vi "WPI_RobotDriveOpen7MotorWithSPARK.vi"(0 "Left Lead Motor":T1=enum."Invalid", 1 "Left Motor Inverted":bool, 5 "Left Follower Motor":T1=enum."Invalid", 7 "Front Left Motor":T1=enum."Invalid", 9 "Front Right Motor":T1=enum."Invalid", 12 "Front Left Motor Inverted":bool) -> (4 "RobotDriveDevRef":T2={"DevStatus"={"status"=FALSE, "code"=0, "source"=""}, "Motors[]"=[], "Square Inputs"=FALSE, "Max Output"=1.0}, 15 "error out":errorcluster)   [LabVIEW 2018]
doc: "Opens a reference to the robot drive for a four-motor robot using Rev Robotics SPARK motor controllers.\n\nThis software is licensed. Open the labview\\readme\\WPI Robotics Library Open Source License.txt file for more information."
uses:
  <vilib>/Rock Robotics/WPI/SafetyOutput/WPI_SafetyOutputConfigMenu.ctl
  <vilib>/Rock Robotics/WPI/RobotDrive/WPI_RobotDriveOpen2MotorWithExistingMotors.vi
  <vilib>/Rock Robotics/WPI/RobotDrive/WPI_RobotDriveDevRef.ctl
  <vilib>/Rock Robotics/WPI/MotorControl/WPI_MotorControlDeviceRef.ctl
  <vilib>/Rock Robotics/SystemInterfaces/DIO/FPGA_DIOChannel.ctl
  <vilib>/Rock Robotics/SystemInterfaces/DIO/FPGA_DIOPWMChannel.ctl
  <vilib>/Rock Robotics/WPI/PWM/WPI_PWMDeadband.ctl
  <vilib>/Rock Robotics/WPI/MotorControl/WPI_MotorControlType.ctl
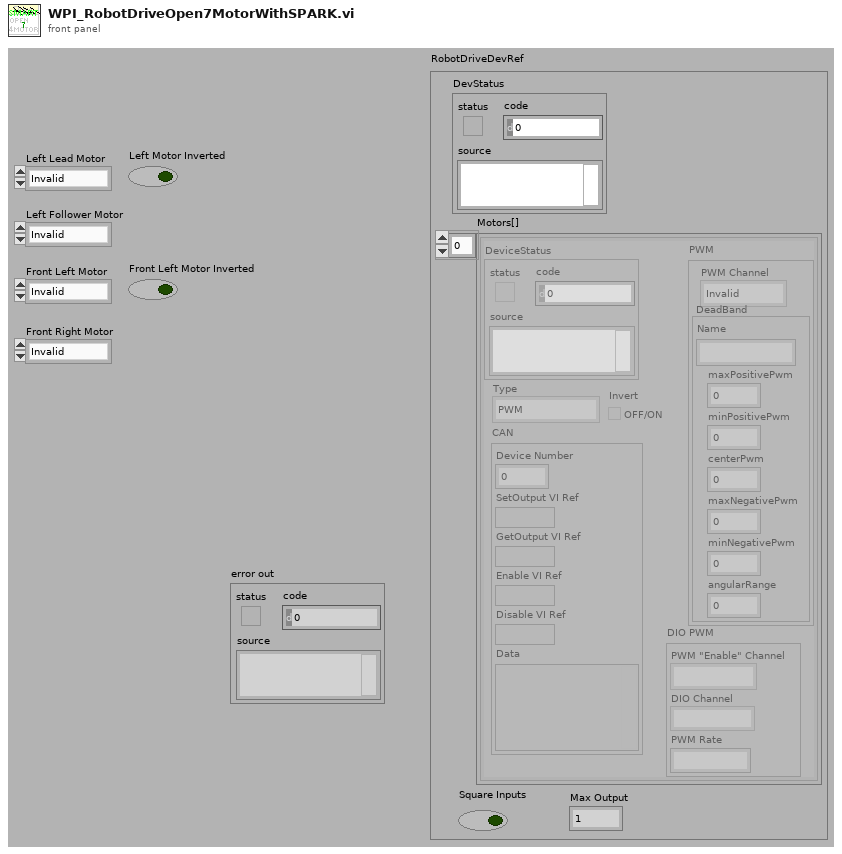
[diagram p1: front panel]
types:
  T1 = typedef "FPGA_DIOPWMChannel.ctl" = enum8{"PWM 0", "PWM 1", "PWM 2", "PWM 3", "PWM 4", "PWM 5", "PWM 6", "PWM 7", "PWM 8", "PWM 9", "PWM MXP 0", "PWM MXP 1", "PWM MXP 2", "PWM MXP 3", "PWM MXP 4", "PWM MXP 5", "PWM MXP 6", "PWM MXP 7", "PWM MXP 8", "PWM MXP 9", "Invalid"}
  T2 = typedef "WPI_RobotDriveDevRef.ctl" = cluster{"DevStatus":errorcluster, "Motors[]":T3[], "Square Inputs":bool, "Max Output":dbl}
  T3 = typedef "WPI_MotorControlDeviceRef.ctl" = cluster{"DeviceStatus":errorcluster, "Type":T4, "PWM":cluster{"PWM Channel":T1, "DeadBand":T5}, "CAN":cluster{"Device Number":u8, "SetOutput VI Ref":variant, "GetOutput VI Ref":variant, "Enable VI Ref":variant, "Disable VI Ref":variant, "Data":variant}, "Invert":bool, "DIO PWM":cluster{"PWM \"Enable\" Channel":T1, "DIOChannel":T6, "PWM Rate":dbl}}
  T4 = typedef "WPI_MotorControlType.ctl" = enum16{"PWM", "CAN", "DIO PWM"}
  T5 = typedef "WPI_PWMDeadband.ctl" = cluster{"Name":string, "maxPositivePwm":i32, "minPositivePwm":i32, "centerPwm":i32, "maxNegativePwm":i32, "minNegativePwm":i32, "angularRange":u16}
  T6 = typedef "FPGA_DIOChannel.ctl" = enum8{"DIO 0", "DIO 1", "DIO 2", "DIO 3", "DIO 4", "DIO 5", "DIO 6", "DIO 7", "DIO 8", "DIO 9", "DIO MXP 0", "DIO MXP 1", "DIO MXP 2", "DIO MXP 3", "DIO MXP 4", "DIO MXP 5", "DIO MXP 6", "DIO MXP 7", "DIO MXP 8", "DIO MXP 9", "DIO MXP 10", "DIO MXP 11", "DIO MXP 12", "DIO MXP 13", "DIO MXP 14", "DIO MXP 15", "SPI Port CS1", "SPI Port CS2", "SPI Port CS3", "SPI Port MISO", "SPI Port MOSI", "Invalid"}
  T7 = typedef "WPI_SafetyOutputConfigMenu.ctl" = enum16{"Enable", "Disable"}
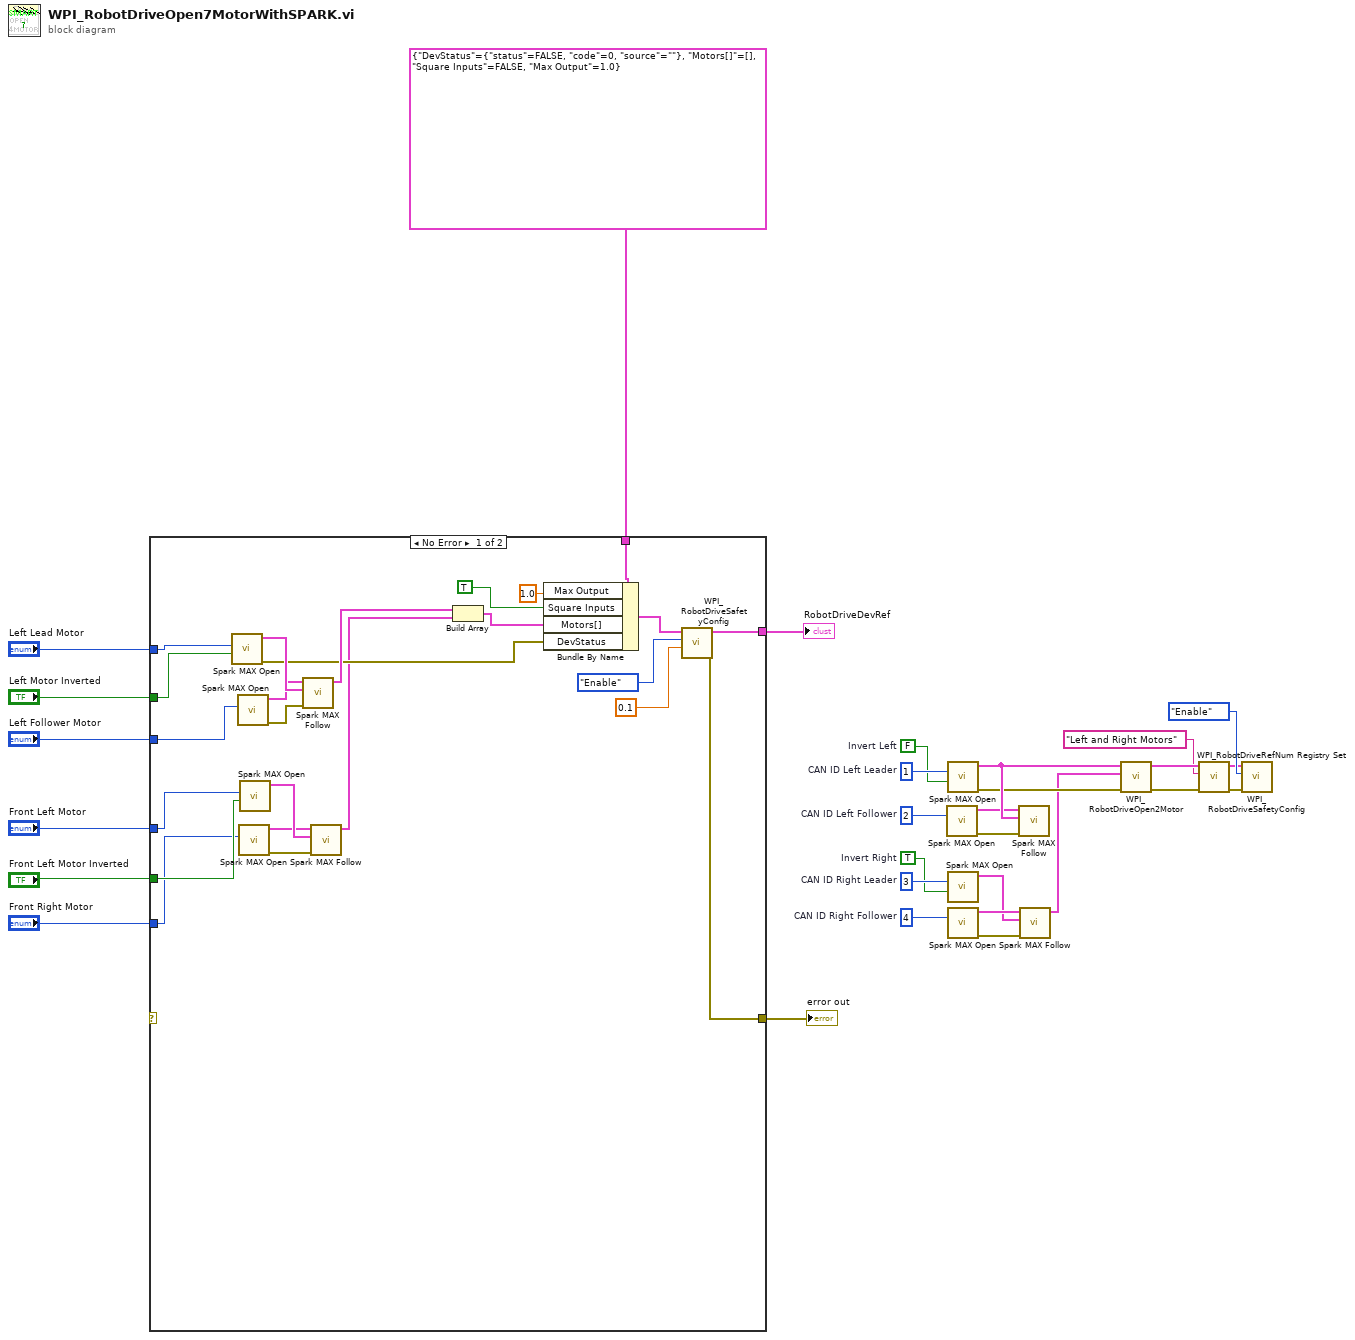
[diagram p0: block diagram]
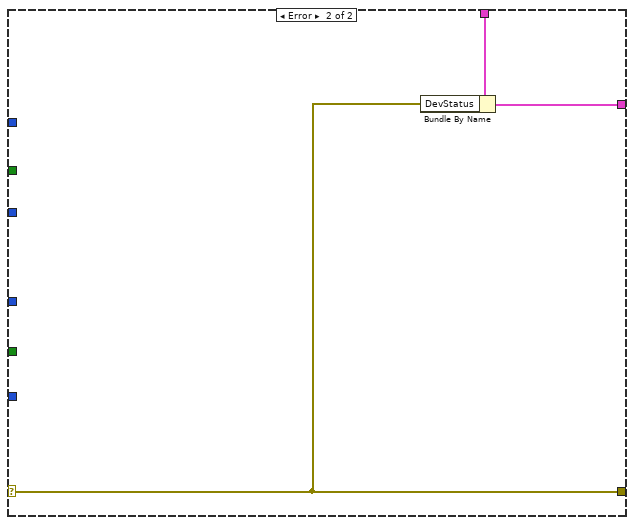
[diagram p2: hidden frame]
diagram:
  w1 = FALSE  # Invert Left
  w2 = TRUE  # Invert Right
  w11 = u8 3  # CAN ID Right Leader
  w10 = u8 4  # CAN ID Right Follower
  w19 = u8 1  # CAN ID Left Leader
  w20 = u8 2  # CAN ID Left Follower
  n1 = case shown="No Error" {
    selector: _ -> [_ w54]
    tunnel: [w48 w55] -> w29
    tunnel: T2 {"DevStatus"={"status"=FALSE, "code"=0, "source"=""}, "Motors[]"=[], "Square Inputs"=FALSE, "Max Output"=1.0} ("RobotDriveDevRef") -> [w53 w56]
    tunnel: "Left Lead Motor" -> [w42 _]
    tunnel: "Front Right Motor" -> [w32 _]
    tunnel: "Front Left Motor" -> [w34 _]
    tunnel: "Left Follower Motor" -> [w40 _]
    tunnel: "Left Motor Inverted" -> [w41 _]
    tunnel: "Front Left Motor Inverted" -> [w33 _]
    tunnel: [w49 w54] -> w22
    frame No Error {
      n2 = call <vilib>:"Spark MAX Open.vi"("Invert"=w41, "Device Number"=w42) -> ("error out"=w38:errorcluster, "MotorControlDeviceRef"=w45:T3)  [unwired: 8 in]
      n3 = call <vilib>:"Spark MAX Open.vi"("Device Number"=w40) -> ("error out"=w43:errorcluster, "MotorControlDeviceRef"=w44:T3)  [unwired: 9 in]
      n4 = call <vilib>:"Spark MAX Open.vi"("Device Number"=w32) -> ("error out"=w35:errorcluster, "MotorControlDeviceRef"=w36:T3)  [unwired: 9 in]
      n5 = call <vilib>:"Spark MAX Open.vi"("Invert"=w33, "Device Number"=w34) -> ("MotorControlDeviceRef"=w37:T3)  [unwired: 8 in, 1 out]
      n6 = call <vilib>:"Spark MAX Follow.vi"("error in (no error)"=w43, "Master Controller"=w45, "MotorControlDeviceRef"=w44) -> ("MotorControlDeviceRef"=w39:T3)  [unwired: 7 in, 1 out]
      n7 = call <vilib>:"Spark MAX Follow.vi"("error in (no error)"=w35, "Master Controller"=w37, "MotorControlDeviceRef"=w36) -> ("MotorControlDeviceRef"=w31:T3)  [unwired: 7 in, 1 out]
      n8 = Build Array(w39, w31) -> (w30:T3[])
      n9 = Bundle By Name(cluster=w53, "Max Output"=1.0, "Square Inputs"=TRUE ("DestroyPWM?"), "Motors[]"=w30, "DevStatus"=w38) -> (w50:T2)
      n10 = call <vilib>:"WPI_RobotDriveSafetyConfig.vi"("timeout (s)"=0.1, "mode"=WPI_SafetyOutputConfigMenu."Enable", "RobotDriveDevRef"=w50) -> ("error out"=w49:errorcluster, "RobotDriveDevRef"=w48:T2)  [unwired: 1 in, 6 out]
    }
    frame Error {
      n11 = Bundle By Name(cluster=w56, "DevStatus"=w54) -> (w55:T2)
    }
  }
  "RobotDriveDevRef" <- w29
  "error out" <- w22
  n12 = call <vilib>:"Spark MAX Open.vi"("Device Number"=w20) -> ("error out"=w15:errorcluster, "MotorControlDeviceRef"=w16:T3)  [unwired: 9 in]
  n13 = call <vilib>:"Spark MAX Open.vi"("Invert"=w1, "Device Number"=w19) -> ("error out"=w17:errorcluster, "MotorControlDeviceRef"=w18:T3)  [unwired: 8 in]
  n14 = call <vilib>:"Spark MAX Open.vi"("Invert"=w2, "Device Number"=w11) -> ("MotorControlDeviceRef"=w12:T3)  [unwired: 8 in, 1 out]
  n15 = call <vilib>:"Spark MAX Open.vi"("Device Number"=w10) -> ("error out"=w14:errorcluster, "MotorControlDeviceRef"=w13:T3)  [unwired: 9 in]
  n16 = call <vilib>:"Spark MAX Follow.vi"("error in (no error)"=w15, "Master Controller"=w18, "MotorControlDeviceRef"=w16) -> ()  [unwired: 7 in, 2 out]
  n17 = call <vilib>:"Spark MAX Follow.vi"("error in (no error)"=w14, "Master Controller"=w12, "MotorControlDeviceRef"=w13) -> ("MotorControlDeviceRef"=w9:T3)  [unwired: 7 in, 1 out]
  n18 = call-poly <vilib>:"WPI_RobotDriveOpen2Motor.vi"("error in (no error)"=w17, "Right Motor Dev Ref"=w9, "Left Motor Dev Ref"=w18) -> ("error out"=w6:errorcluster, "RobotDriveDevRef"=w8:T2)  [unwired: 7 in]
  n19 = call <vilib>:"WPI_RobotDriveRefNum Registry Set.vi"("error in (no error)"=w6, "refnum name"="Left and Right Motors", "RobotDriveDevRef"=w8) -> ("error out"=w3:errorcluster, "RobotDriveDevRef"=w4:T2)  [unwired: 7 in]
  n20 = call <vilib>:"WPI_RobotDriveSafetyConfig.vi"("error in (no error)"=w3, "mode"=WPI_SafetyOutputConfigMenu."Enable", "RobotDriveDevRef"=w4) -> ()  [unwired: 7 in, 2 out]
